vi "GetMaxAndMinPriorities.vi"(8 "error in":errorcluster, 11 "queues in":refnum<class "CLM_PriorityLocalMessage.lvclass">) -> (0 "error out":errorcluster, 1 "lowest priority":i32, 2 "highest priority":i32, 3 "queues out":refnum<class "CLM_PriorityLocalMessage.lvclass">)   [LabVIEW 2013, in "CLM_PriorityLocalMessage.lvclass"]
uses:
  CLM_PriorityLocalMessage.lvclass
  CLM_PriorityLocalMessage.lvclass/CLM_PriorityLocalMessage.ctl
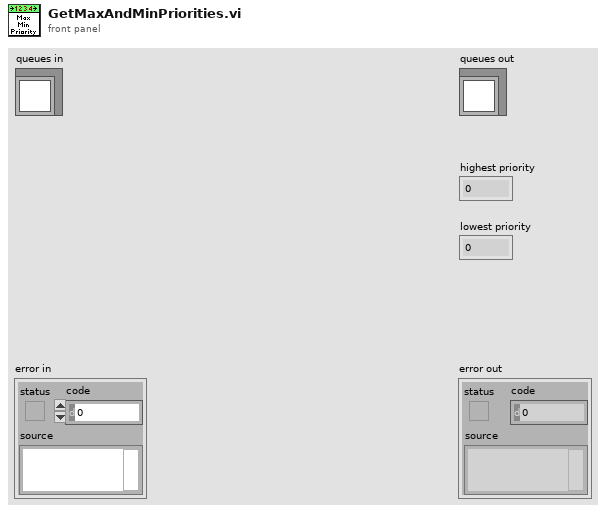
[diagram p1: front panel]
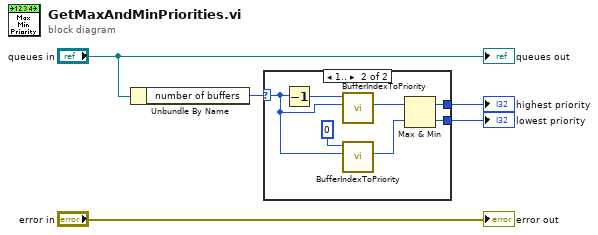
[diagram p0: block diagram]
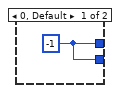
[diagram p2: hidden frame]
diagram:
  n1 = Unbundle By Name("queues in") -> ("number of buffers"=w1:i32)
  n2 = case shown="1.." w1 {
    selector: w1 -> [_ w7]
    tunnel: [w6 w9] -> w3
    tunnel: [w6 w8] -> w2
    frame 0, Default {
      w6 = -1
    }
    frame 1.. {
      n3 = Decrement(x=w7) -> (x-1=w10:i32)
      n4 = call "BufferIndexToPriority.vi"("number of buffers"=w7, "buffer index"=w10) -> ("priority"=w12:i32)  [unwired: 6 in, 3 out]
      n5 = call "BufferIndexToPriority.vi"("number of buffers"=w7, "buffer index"=0) -> ("priority"=w11:i32)  [unwired: 6 in, 3 out]
      n6 = Max & Min(x=w12, y=w11) -> (max(x,y)=w9:i32, min(x,y)=w8:i32)
    }
  }
  "highest priority" <- w3
  "lowest priority" <- w2
  "error out" <- "error in"
  "queues out" <- "queues in"
